vi "TEST BUTTON PRESS.vi"() -> ()   [LabVIEW 2023]
panel:
  in  "stop":bool
  out "Boolean 2":bool
  in  "Boolean":bool
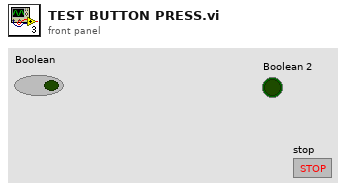
[diagram p1: front panel]
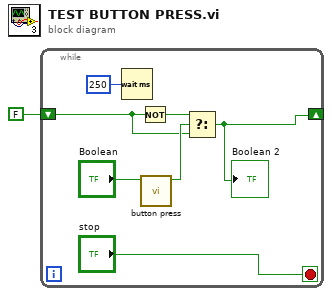
[diagram p0: block diagram]
diagram:
  n1 = while {
    shift-right: [w4] -> _
    shift-left: FALSE -> [w3]
    stop <- "stop" stop-if-true
    n2 = Wait (ms)(milliseconds to wait=u32 250) -> ()  [unwired: 1 out]
    n3 = Not(x=w3) -> (.not. x?=w2:bool)
    n4 = call "button press.vi"("button IN"="Boolean") -> ("Button Pressed?"=w5:bool)  [unwired: 10 in]
    n5 = Select(t=w2, s=w5, f=w3) -> (s? t:f=w4:bool)
    "Boolean 2" <- w4
  }
